vi "libssh2_sftp_read.vi"(8 "error in (no error)":errorcluster, 10 "buffer maxlen":i32, 11 "sftp handle":T1) -> (0 "error out":errorcluster, 1 "bytes read":i64, 2 "buffer":u8[](array[numeric]))   [LabVIEW 2017, in "libssh2.lvlib"]
doc: "Read data from a file handle."
uses:
  libssh2.lvlib
  SFTP Handle Refnum.ctl
  Acquire SFTP.vi
  Release SFTP.vi
  Acquire Session.vi
  Release Session.vi
  Not An SFTP Handle Refnum.vi
  <vilib>/Utility/error.llb/Error Cluster From Error Code.vi
  Global Settings.vi
  Read SFTP Handle Refnum.vi
  Read SFTP Refnum.vi
  Read Session Refnum.vi
  <vilib>/Utility/semaphor.llb/Acquire Semaphore.vi
  <vilib>/Utility/semaphor.llb/Release Semaphore.vi
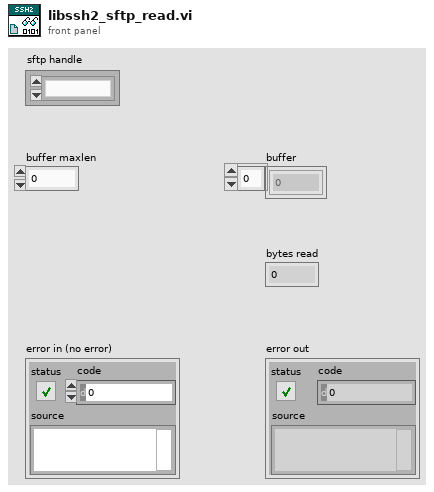
[diagram p1: front panel]
types:
  T1 = typedef "libssh2.lvlib/SFTP Handle Refnum.ctl" = refnum<k1>
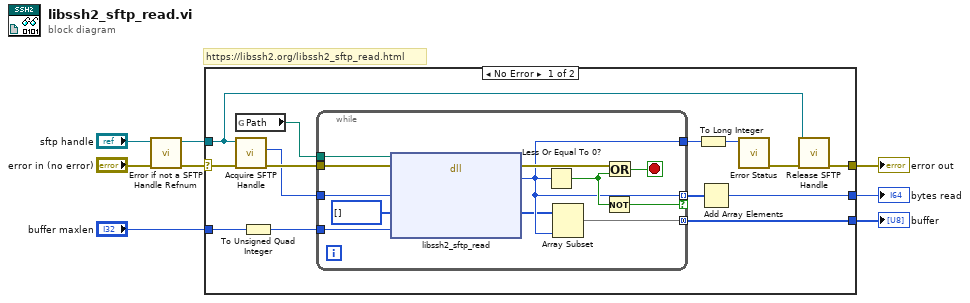
[diagram p0: block diagram]
diagram:
  # "https://libssh2.org/libssh2_sftp_read.html"
  n1 = call "Error if not a SFTP Handle Refnum.vi"("error in (no error)"="error in (no error)", "sftp handle"="sftp handle") -> ("error out"=w7:errorcluster, "sftp handle out"=w6:T1)  [unwired: 8 in]
  n2 = case shown="No Error" w7 {
    selector: w7 -> [w21 w35]
    tunnel: w6 -> [w10 _]
    tunnel: [w11 w35] -> w5
    tunnel: "buffer maxlen" -> [w16 _]
    tunnel: [w13 _] -> w2
    tunnel: [w9 _] -> w1
    frame No Error {
      n3 = global read "Global Settings.vi" "Path"() -> (w22:path)
      n4 = call "Acquire SFTP Handle.vi"("error in (no error)"=w21, "sftp handle"=w10) -> ("error out"=w20:errorcluster, "LIBSSH2_SFTP_HANDLE*"=w19:u64)  [unwired: 8 in]
      n5 = To Unsigned Quad Integer(1:w16) -> (0:w15:u64)
      n6 = while {
        tunnel: w22 -> [w34]
        tunnel: w20 -> [w26]
        tunnel: w19 -> [w33]
        tunnel: [w25] -> w17
        tunnel: w15 -> [w29]
        tunnel: [w25] -> w14 mode=indexing if=w31
        tunnel: [w23] -> w9 mode=concatenating
        stop <- w32 stop-if-true
        n7 = dll-call lib="?" fn="libssh2_sftp_read"(path in=w34, error in=w26, "handle"=w33, "buffer"=u8[] [], "buffer_maxlen"=w29) -> (error out=w28:errorcluster, "return value"=w25:i64, "buffer"=w24:u8[])  [unwired: 3 in, 1 out]
        n8 = Less Or Equal To 0?(x=w25) -> (x <= 0?=w30:bool)
        n9 = Array Subset(array=w24, length=w25) -> (w23:u8[])  [unwired: 1 in]
        n10 = Not(x=w30) -> (.not. x?=w31:bool)
        n11 = Or(x=w28, y=w30) -> (x .or. y?=w32:bool)
      }
      n12 = To Long Integer(number=w17) -> (32bit integer=w12:i32)
      n13 = Add Array Elements(numeric array=w14) -> (sum=w13:i64)
      n14 = call "Error Status.vi"("return value"=w12) -> ("error out"=w18:errorcluster)  [unwired: 9 in, 1 out]
      n15 = call "Release SFTP Handle.vi"("error in (no error)"=w18, "sftp handle"=w10) -> ("error out"=w11:errorcluster)  [unwired: 9 in]
    }
    frame Error {
    }
  }
  "error out" <- w5
  "bytes read" <- w2
  "buffer" <- w1
